vi "UTILITY Boolean Event.vi"(7 "Status":T1, 8 "error in (no error)":errorcluster, 10 "Set Status":bool, 11 "name (unnamed)":string) -> (0 "error out":errorcluster, 3 "latest READ notification":bool)   [LabVIEW 2014]
uses:
  Type Definitions/UTILITY Notifier.ctl
panel:
  out "user event out":refnum<user-event>
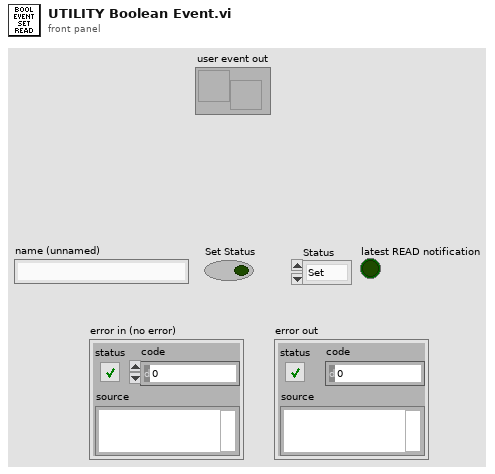
[diagram p1: front panel]
types:
  T1 = typedef "UTILITY Notifier.ctl" = enum16{"Set", "Read", "Release Ref"}
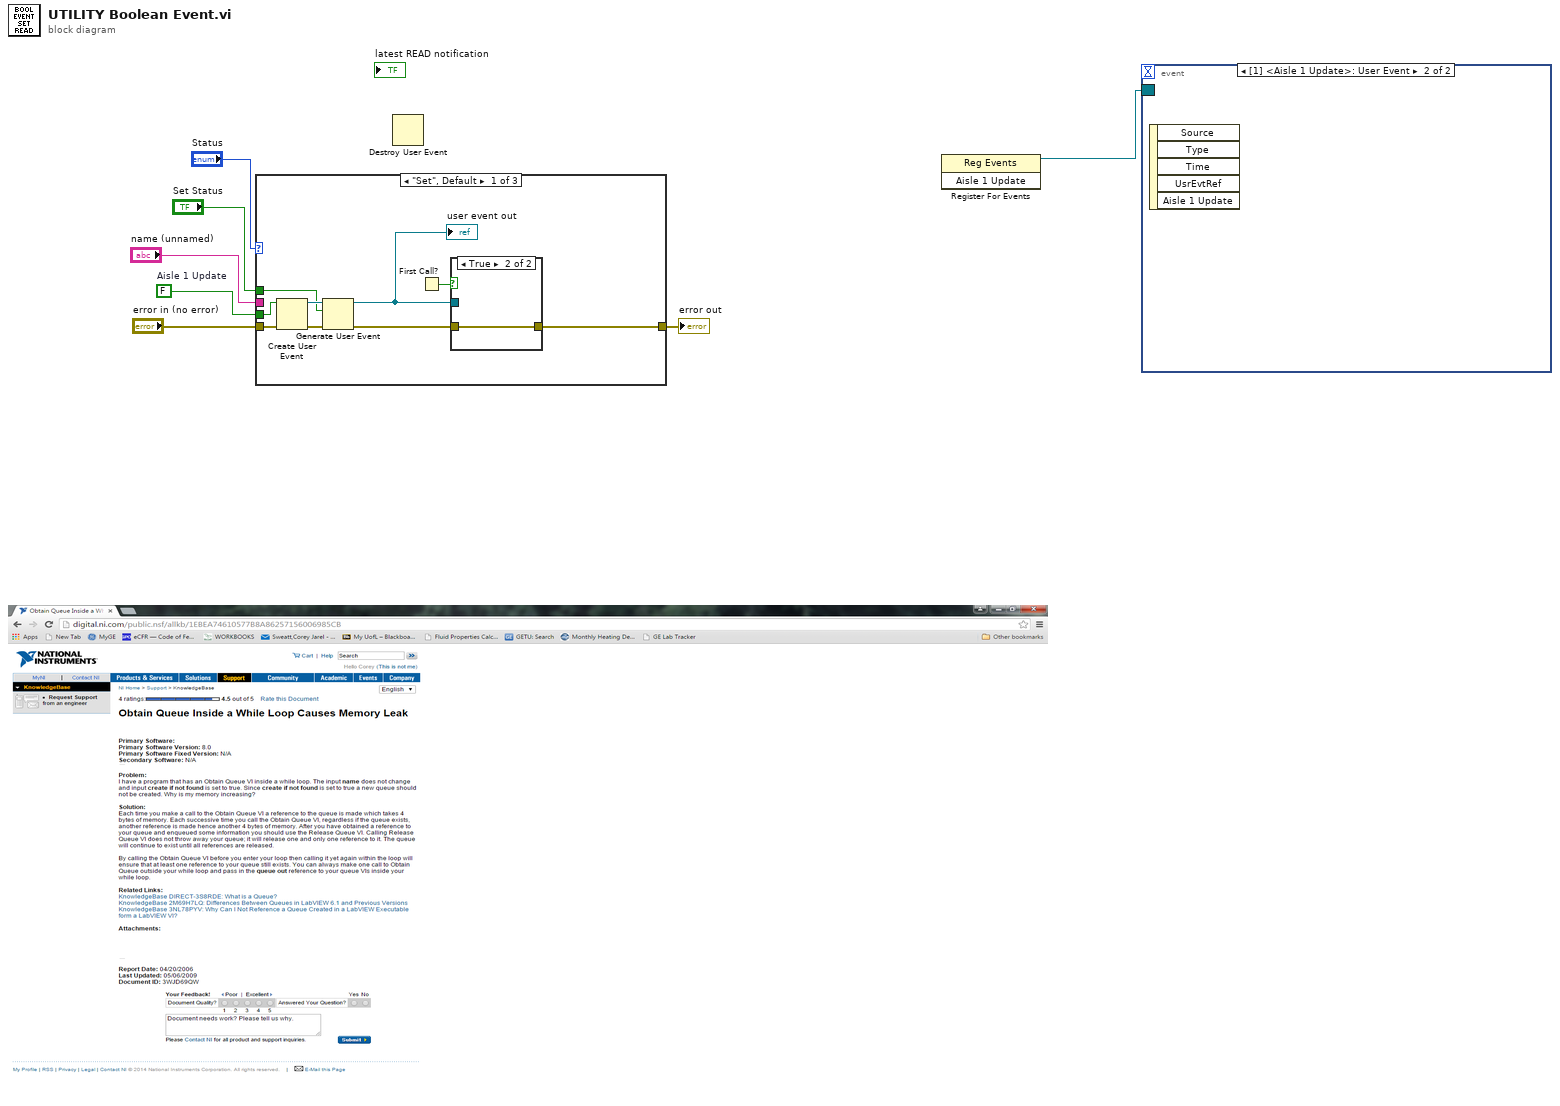
[diagram p0: block diagram]
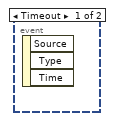
[diagram p2: hidden frame]
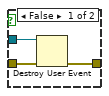
[diagram p3: hidden frame]
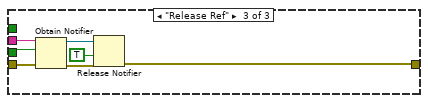
[diagram p5: hidden frame]
diagram:
  w2 = FALSE  # Aisle 1 Update
  n1 = case shown="\"Set\", Default" "Status" {
    tunnel: [w16 _ w22] -> w7
    tunnel: "error in (no error)" -> [w13 _ w27]
    tunnel: "name (unnamed)" -> [_ _ w25]
    tunnel: "Set Status" -> [w9 _ _]
    tunnel: w2 -> [w14 _ w24]
    frame "Set", Default {
      n2 = Create User Event(user event datatype=w14, error in=w13) -> (user event=w10:refnum<user-event>, error out=w12:errorcluster)
      n3 = Generate User Event(user event=w10, event data cluster=w9, error in=w12) -> (user event out=w8:refnum<user-event>, error out=w11:errorcluster)  [unwired: 1 in]
      "user event out" <- w8
      n4 = First Call?() -> (First Call?: T/F=w15:bool)
      n5 = case shown="True" w15 {
        tunnel: w11 -> [w18 w20]
        tunnel: [w17 w20] -> w16
        tunnel: w8 -> [w19 _]
        frame False {
          n6 = Destroy User Event(user event=w19, error in=w18) -> (error out=w17:errorcluster)
        }
        frame True {
        }
      }
    }
    frame "Read" {
    }
    frame "Release Ref" {
      n7 = Obtain Notifier(name (unnamed)=w25, notification data type=w24, error in (no error)=w27) -> (notifier out=w23:refnum<notifier>, error out=w26:errorcluster)  [unwired: 1 in, 1 out]
      n8 = Release Notifier(notifier=w23, force destroy? (F)=TRUE, error in (no error)=w26) -> (error out=w22:errorcluster)  [unwired: 2 out]
    }
  }
  "error out" <- w7
  n9 = Destroy User Event() -> ()  [unwired: 2 in, 1 out]
  n10 = register-events() -> (reference out=w1:refnum<event-registration>)  [unwired: 3 in, 1 out]
  n11 = event shown="[1] <Aisle 1 Update>: User Event" {
    selector: w1 -> [_ _]
    dyn-events: _ -> [_ _]
    timeout: _ -> [_ _]
    event Timeout {
      n12 = event-data() -> ()  [unwired: 1 in, 3 out]
    }
    event User Event {
      n13 = event-data() -> ()  [unwired: 1 in, 5 out]
    }
  }
